vi "to INT8.vi"(8 "error in":errorcluster, 11 "byte":u8[](array[numeric]) format="%b") -> (0 "error out":errorcluster, 3 "INT8":i8)   [LabVIEW 2020, in "wamplv.lvlib" / "MessagePack.lvclass"]
uses:
  MessagePack.lvclass
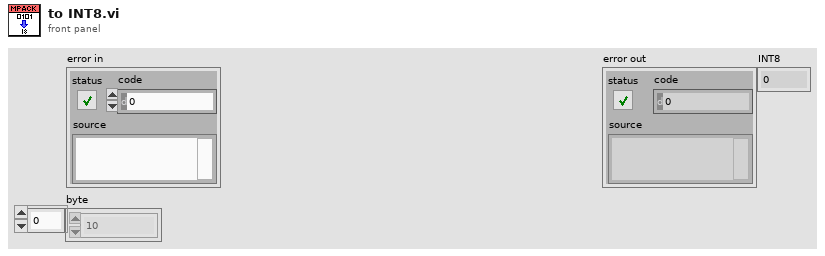
[diagram p1: front panel]
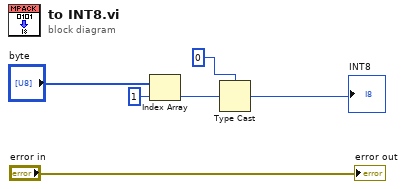
[diagram p0: block diagram]
diagram:
  n1 = Index Array(array="byte", index=1) -> (element=w3:u8)
  n2 = Type Cast(type=i8 0 ("INT8"), x=w3) -> (*(type *) &x=→"INT8":i8)
  "error out" <- "error in"
